vi "PlotPoints.vi"(10 "Array":dbl[][](array[numeric])) -> (2 "XY Graph":cluster{"Array":dbl[], "Array 3":dbl[]}(graph))   [LabVIEW 2017]
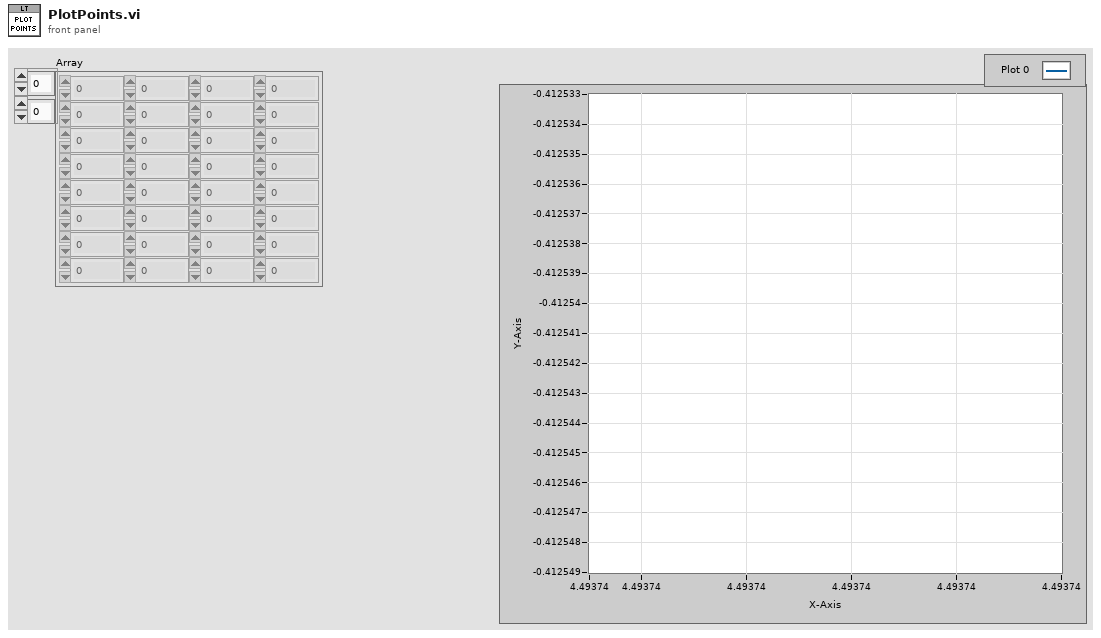
[diagram p1: front panel]
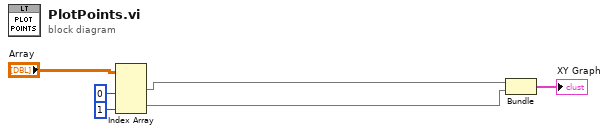
[diagram p0: block diagram]
diagram:
  n1 = Index Array(array="Array", index (col) #1=0 ("disabled index (col)"), index (col) #2=1 ("index (col)")) -> (element #1=w3:dbl[], element #2=w2:dbl[])  [unwired: 2 in]
  n2 = Bundle("Array"=w3, "Array"=w2) -> (→"XY Graph":cluster{"Array":dbl[], "Array":dbl[]})  [unwired: 1 in]
